vi "Configure Noise Tolerance.vi"(8 "error in (no error)":errorcluster, 9 "Noise Tolerance (1.000000E+0)":dbl=1.0 format="%.6e", 10 "Measurement Function (0: Voltage)":i32(ring) items=["Voltage", "Current", "Resistance", "Charge"], 11 "VISA resource name":refnum<visa-resource-name>) -> (0 "error out":errorcluster, 3 "VISA resource name out":refnum<visa-resource-name>)   [LabVIEW 2016, in "Keithley 6517.lvlib"]
doc: "Configures the noise tolerance settings for the measurement functions (Voltage, Current, Resistance and Charge). It's used to set the window when the filter type is Advanced that configured by <b>Configure Average.vi.</b>\n\nNote:\nThe specified measurement should be enabled from <b>Configure Measurement Function.vi</b>.\n\nThis VI is <B>NOT</B> compatible with model <B>6514</B>."
uses:
  <instrlib>/Keithley 6517/Keithley 6517.lvlib
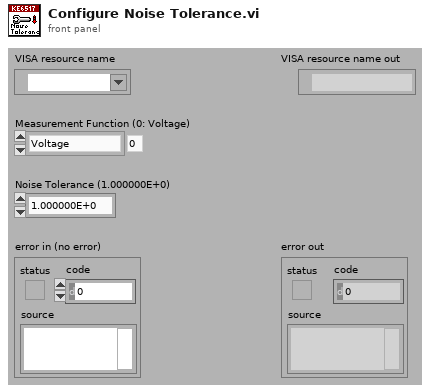
[diagram p1: front panel]
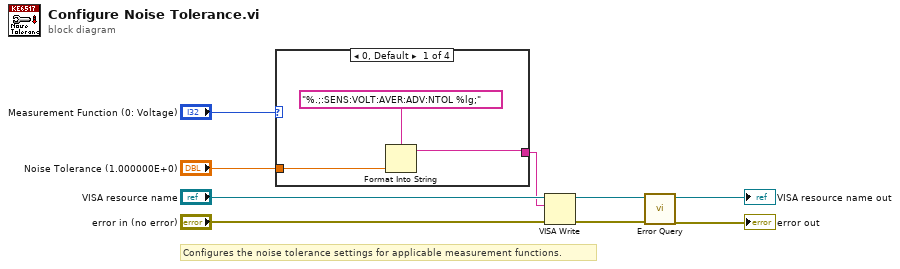
[diagram p0: block diagram]
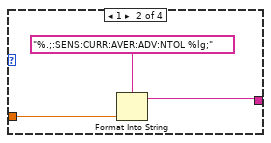
[diagram p2: hidden frame]
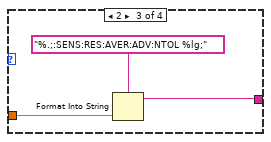
[diagram p3: hidden frame]
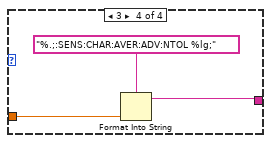
[diagram p4: hidden frame]
diagram:
  # "Configures the noise tolerance settings for applicable measurement functions."
  n1 = case shown="0, Default" "Measurement Function (0: Voltage)" {
    tunnel: "Noise Tolerance (1.000000E+0)" -> [w11 w14 w17 w20]
    tunnel: [w10 w13 w16 w19] -> w1
    frame 0, Default {
      n2 = Format Into String(format string="%.;:SENS:VOLT:AVER:ADV:NTOL %lg;", w11) -> (resulting string=w10:string)  [unwired: 2 in, 1 out]
    }
    frame 1 {
      n3 = Format Into String(format string="%.;:SENS:CURR:AVER:ADV:NTOL %lg;", w14) -> (resulting string=w13:string)  [unwired: 2 in, 1 out]
    }
    frame 2 {
      n4 = Format Into String(format string="%.;:SENS:RES:AVER:ADV:NTOL %lg;", w17) -> (resulting string=w16:string)  [unwired: 2 in, 1 out]
    }
    frame 3 {
      n5 = Format Into String(format string="%.;:SENS:CHAR:AVER:ADV:NTOL %lg;", w20) -> (resulting string=w19:string)  [unwired: 2 in, 1 out]
    }
  }
  n6 = VISA Write(VISA resource name="VISA resource name", write buffer=w1, error in (no error)="error in (no error)") -> (VISA resource name out=w7:refnum<visa-resource-name>, error out=w6:errorcluster)  [unwired: 1 out]
  n7 = call <instrlib>:"Error Query.vi"("error in (no error)"=w6, "VISA resource name"=w7) -> ("error out"=→"error out":errorcluster, "VISA resource name out"=→"VISA resource name out":refnum<visa-resource-name>)  [unwired: 6 in, 2 out]
